vi "AcquireWaveformsFpga.vi"(8 "error in (no error)":errorcluster, 11 "MCSA Acquisition Config":T1 {"FixedSizeX31"."InputConfig" items=["AC Coupled", "DC Coupled", "IEPE AC Coupled"]}) -> (0 "error out":errorcluster, 3 "Waveforms":waveform(sgl)[](array[waveform]))   [LabVIEW 2017, in "McsaFpgaAcquisition.lvlib"]
uses:
  <vilib>/addons/InsightCM/Devices/Shared/Mcsa/McsaFpgaAcquisition/McsaFpgaAcquisition.lvlib
  <vilib>/addons/InsightCM/Devices/Shared/Mcsa/McsaFpgaAcquisition/controls/Configuration.ctl
  <vilib>/addons/InsightCM/Devices/Shared/Cms/CmsAcquisition/controls/FixedSizeArrays.ctl
  <vilib>/LabVIEW Targets/FPGA/cRIO/shared/nicrio_ModuleControls/nicrio_cRIO-9232_ConfigModeRing.ctl
  <vilib>/addons/InsightCM/Devices/Shared/Cms/cRIOWfmAcq/subVIs/RIO Wfm Cust Ctrls/rwfm_SamplingInfo.ctl
  <vilib>/addons/InsightCM/Devices/Shared/Mcsa/McsaFpgaAcquisition/controls/Group.ctl
  <vilib>/addons/InsightCM/Devices/Shared/Mcsa/McsaFpgaAcquisition/controls/ChannelMcsa.ctl
  <vilib>/addons/InsightCM/Devices/Shared/Mcsa/McsaFpgaAcquisition/controls/RangeParams.ctl
  <vilib>/addons/InsightCM/Devices/Shared/Mcsa/cRIOWfmAcqMcsa/cRIOWfmLibMcsa.lvlib
  <vilib>/addons/InsightCM/Utilities/ChannelStatus/ChannelStatus.lvlib
  <vilib>/addons/InsightCM/Devices/Shared/Cms/cRIOWfmAcq/cRIOWfmLib.lvlib
  <vilib>/addons/InsightCM/Devices/Shared/Cms/CmsAcquisition/CmsAcquisition.lvlib
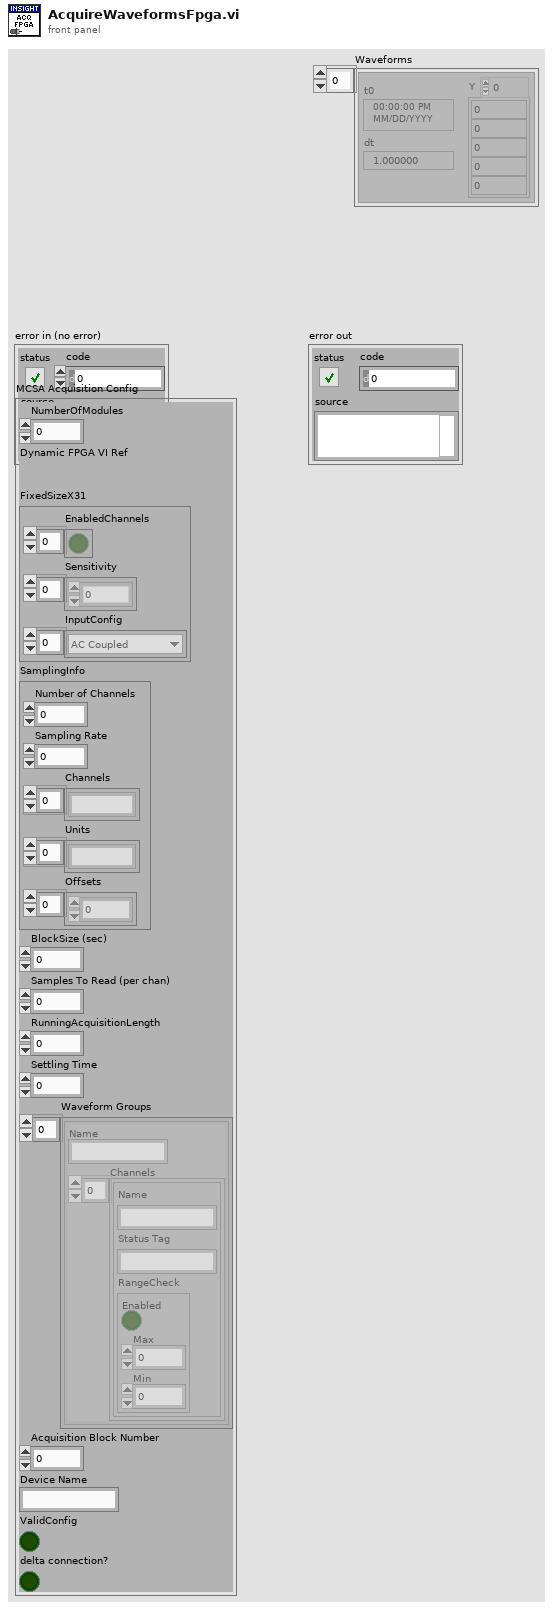
[diagram p1: front panel]
types:
  T1 = typedef "McsaFpgaAcquisition.lvlib/Configuration.ctl" = cluster{"NumberOfModules":i16, "Dynamic FPGA VI Ref":refnum<k20>, "FixedSizeX31":T2, "SamplingInfo":T4, "BlockSize (sec)":dbl, "Samples To Read (per chan)":i32, "RunningAcquisitionLength":dbl, "Settling Time":dbl, "Waveform Groups":T5[], "Acquisition Block Number":i32, "Device Name":string, "ValidConfig":bool, "delta connection?":bool}
  T2 = typedef "CmsAcquisition.lvlib/FixedSizeArrays.ctl" = cluster{"EnabledChannels":bool[], "Sensitivity":dbl[], "InputConfig":T3[]}
  T3 = typedef "nicrio_cRIO-9232_ConfigModeRing.ctl" = u8
  T4 = typedef "cRIOWfmLib.lvlib/rwfm_SamplingInfo.ctl" = cluster{"Number of Channels":i32, "Sampling Rate":dbl, "Channels":string[], "Units":string[], "Offsets":sgl[]}
  T5 = typedef "McsaFpgaAcquisition.lvlib/Group.ctl" = cluster{"Name":string, "Channels":T6[]}
  T6 = typedef "McsaFpgaAcquisition.lvlib/ChannelMcsa.ctl" = cluster{"Name":string, "Status Tag":string, "RangeCheck":T7}
  T7 = typedef "McsaFpgaAcquisition.lvlib/RangeParams.ctl" = cluster{"Enabled":bool, "Max":dbl, "Min":dbl}
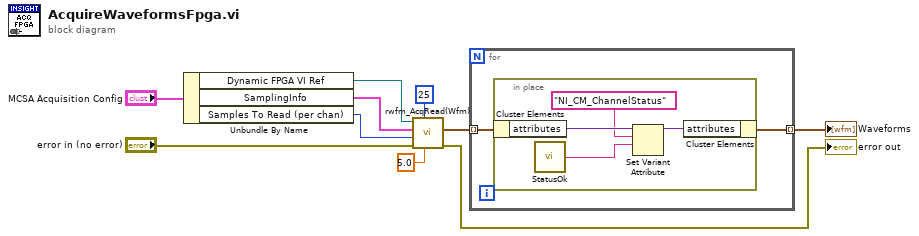
[diagram p0: block diagram]
diagram:
  n1 = Unbundle By Name("MCSA Acquisition Config") -> ("Dynamic FPGA VI Ref"=w6:refnum<k20>, "SamplingInfo"=w5:T4, "Samples To Read (per chan)"=w4:i32)
  n2 = call <vilib>:"rwfm_AcqRead(Wfm).vi"("Timeout (s)"=5.0, "Poll Time (ms)"=u32 25, "error in"="error in (no error)", "Samps Read per Chan"=w4, "Sampling Info"=w5, "Dynamic FPGA VI Reference"=w6) -> ("error out"=→"error out":errorcluster, "Wfm Data"=w3:waveform(sgl)[])  [unwired: 4 out]
  n3 = for {
    tunnel: w3 -> [w12] mode=indexing
    tunnel: [w11] -> w2 mode=indexing
    n4 = in-place {
      n5 = in-place-cluster #1(w12) -> ("attributes"=w16:variant)
      n6 = call <vilib>:"StatusOk.vi"() -> ("status"=w13:string)  [unwired: 5 in]
      n7 = Set Variant Attribute(Variant=w16, name="NI_CM_ChannelStatus", value=w13) -> (Variant out=w15:variant)  [unwired: 1 in, 2 out]
      n8 = in-place-cluster #1("attributes"=w15) -> (w11:waveform(sgl))
    }
  }
  "Waveforms" <- w2
